vi "Wait ms.vi"(8 "error in (no error)":errorcluster, 11 "milliseconds to wait":u32) -> (0 "error in (no error) 2":errorcluster)   [LabVIEW 2021]
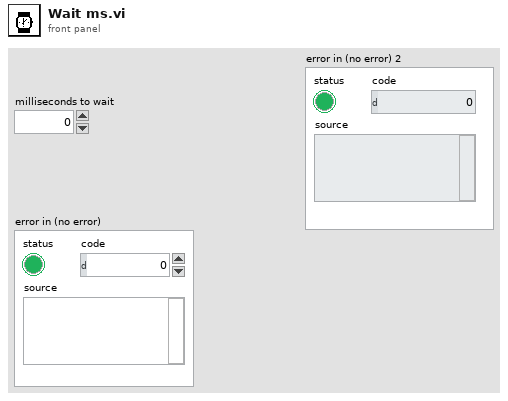
[diagram p1: front panel]
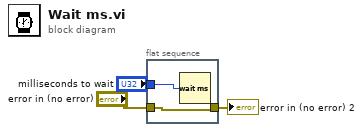
[diagram p0: block diagram]
diagram:
  n1 = flat-sequence {
    tunnel: "error in (no error)" -> [w5]
    tunnel: [w5] -> w1
    tunnel: "milliseconds to wait" -> [w4]
    frame #0 {
      n2 = Wait (ms)(milliseconds to wait=w4) -> ()  [unwired: 1 out]
    }
  }
  "error in (no error) 2" <- w1
